vi "MGI Symbolic To Path.vi"(10 "Symbolic Path":path) -> (1 "Symbolic Folder":T1, 2 "Symbolic?":bool, 3 "Path":path)   [LabVIEW 2020]
doc: "Build an absolute path from <B>Start</B> and <B>Rel Path</B>. <B>Start</B> may be a symbolic name such as \"Desktop\".\n\nAuthored by Shawn Walpole\nsupport@mooregoodideas.com\nwww.mooregoodideas.com\n\nCopyright (c) 2013, Moore Good Ideas, Inc.\n\nAll rights reserved.\n\nRedistribution and use in source and binary forms, with or without modification, are permitted provided that the following conditions are met:\n\n * Redistributions of source code must retain the above copyright notice, this list of conditions and the following disclaimer.\n * Redistributions in binary form must reproduce the above copyright notice, this list of conditions and the following disclaimer in the documentation and/or other materials provided with the distribution.\n * Neither the name of Moore Good Ideas, Inc. nor the names of its contributors may be used to endorse or promote products derived from this software without specific prior written permission.\n\nTHIS SOFTWARE IS PROVIDED BY THE COPYRIGHT HOLDERS AND CONTRIBUTORS \"AS IS\" AND ANY EXPRESS OR IMPLIED WARRANTIES, INCLUDING, BUT NOT LIMITED TO, THE IMPLIED WARRANTIES OF MERCHANTABILITY AND FITNESS FOR A PARTICULAR PURPOSE ARE DISCLAIMED. IN NO EVENT SHALL THE COPYRIGHT OWNER OR CONTRIBUTORS BE LIABLE FOR ANY DIRECT, INDIRECT, INCIDENTAL, SPECIAL, EXEMPLARY, OR CONSEQUENTIAL DAMAGES (INCLUDING, BUT NOT LIMITED TO, PROCUREMENT OF SUBSTITUTE GOODS OR SERVICES; LOSS OF USE, DATA, OR PROFITS; OR BUSINESS INTERRUPTION) HOWEVER CAUSED AND ON ANY THEORY OF LIABILITY, WHETHER IN CONTRACT, STRICT LIABILITY, OR TORT (INCLUDING NEGLIGENCE OR OTHERWISE) ARISING IN ANY WAY OUT OF THE USE OF THIS SOFTWARE, EVEN IF ADVISED OF THE POSSIBILITY OF SUCH DAMAGE."
uses:
  <userlib>/_MGI/File/MGI Windows Folder Enum.ctl
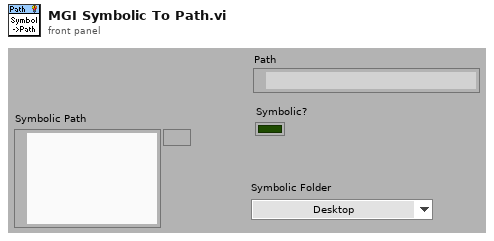
[diagram p1: front panel]
types:
  T1 = typedef "MGI Windows Folder Enum.ctl" = enum32{"Desktop", "Err<Internet>", "Programs", "Err<Controls>", "Err<Printers>", "Personal (MyDocuments)", "Favorites", "Startup", "Recent", "SendTo", "Err<RecycleBin>", "StartMenu", "Err<MyDocuments>", "MyMusic", "MyVideo", "Err<0x000F>", "DesktopDirectory", "Err<Drives>", "Err<Network>", "NetHood", "Fonts", "Templates", "CommonStartMenu", "CommonPrograms", "CommonStartup", "CommonDesktopDirectory", "AppData", "PrintHood", "LocalAppData", "Err<AltStartup>", "Err<CommonAltStartup>", "CommonFavorites", "InternetCache", "Cookies", "History", "CommonAppData", "Windows", "System", "ProgramFiles", "MyPictures", "Profile", "System32", "Err<0x002A>", "ProgramFilesCommon", "Err<0x002C>", "CommonTemplates", "CommonDocuments", "CommonAdminTools", "AdminTools"}
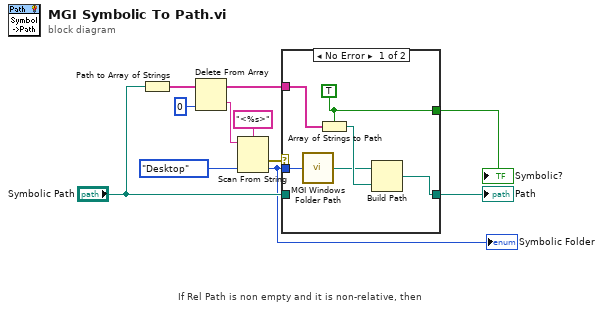
[diagram p0: block diagram]
diagram:
  # "If Rel Path is non empty and it is non-relative, then"
  n1 = Path to Array of Strings(0:"Symbolic Path") -> (2:w11:string[])  [unwired: 1 out]
  n2 = Delete From Array(array=w11, index=0) -> (deleted portion=w10:string, array with subset deleted=w7:string[])  [unwired: 1 in]
  n3 = Scan From String(format string="<%s>", input string=w10, default 1=MGI_Windows_Folder_Enum."Desktop" ("Windows Folder")) -> (error out=w9:errorcluster, output 1=w5:T1)  [unwired: 2 in, 2 out]
  "Symbolic Folder" <- w5
  n4 = case shown="No Error" w9 {
    tunnel: "Symbolic Path" -> [_ w18]
    tunnel: w5 -> [w13 _]
    tunnel: w7 -> [w17 _]
    tunnel: [w15 w18] -> w6
    tunnel: [w14 _] -> w4
    frame No Error {
      w14 = TRUE ("relative")
      n5 = call <userlib>:"MGI Windows Folder Path.vi"("Windows Folder"=w13) -> ("Path"=w12:path)
      n6 = Array of Strings to Path(0:w17, 1:w14) -> (2:w16:path)
      n7 = Build Path(base path=w12, name or relative path=w16) -> (appended path=w15:path)
    }
    frame Error {
    }
  }
  "Path" <- w6
  "Symbolic?" <- w4
